vi "asdfasdfa.vi"(11 "cluster":T1) -> (3 "x/y":dbl)   [LabVIEW 2021]
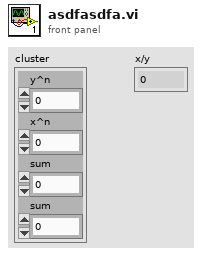
[diagram p1: front panel]
types:
  T1 = cluster{"y^n":dbl, "x^n":dbl, "sum":dbl, "sum":dbl}
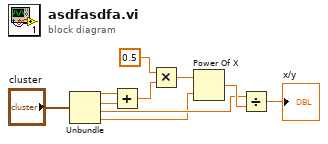
[diagram p0: block diagram]
diagram:
  n1 = Unbundle("cluster") -> ("y^n"=w1:dbl, "x^n"=w2:dbl, "sum"=w7:dbl, "sum"=w5:dbl)
  n2 = Add(x=w1, y=w2) -> (x+y=w4:dbl)
  n3 = Multiply(x=0.5, y=w4) -> (x*y=w6:dbl)
  n4 = Power Of X(1:w5, 2:w6) -> (0:w8:dbl)
  n5 = Divide(x=w7, y=w8) -> (x/y=→"x/y":dbl)
